vi "get all VIs in SciScan directory.vi"(7 "Path":path, 11 "keep GFG unlocked":bool) -> (3 "All Files in Dir":path[](array[path]))   [LabVIEW 2012]
doc: "SciScan 1.2 160622"
panel:
  out "size(s)":i32
  out "error out":errorcluster
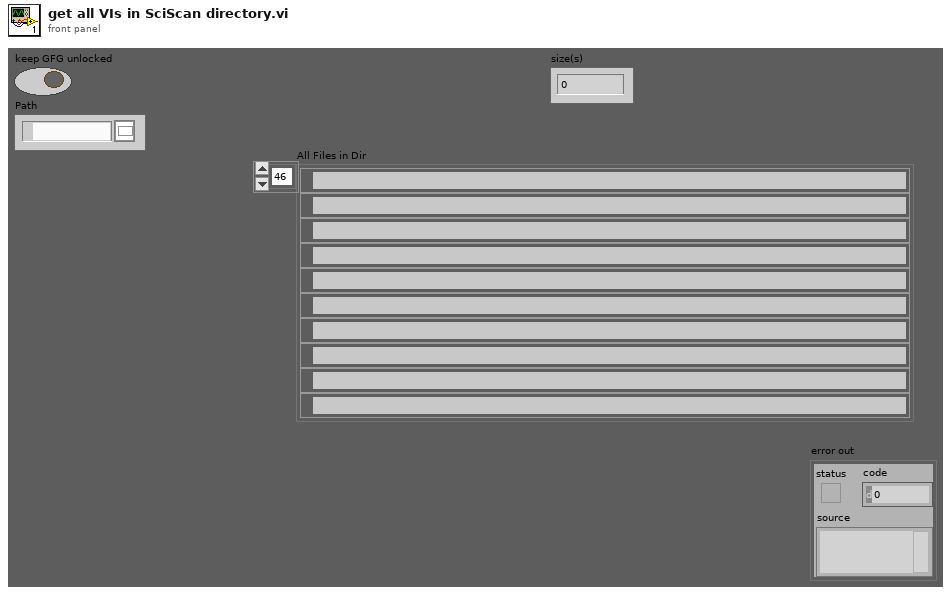
[diagram p1: front panel]
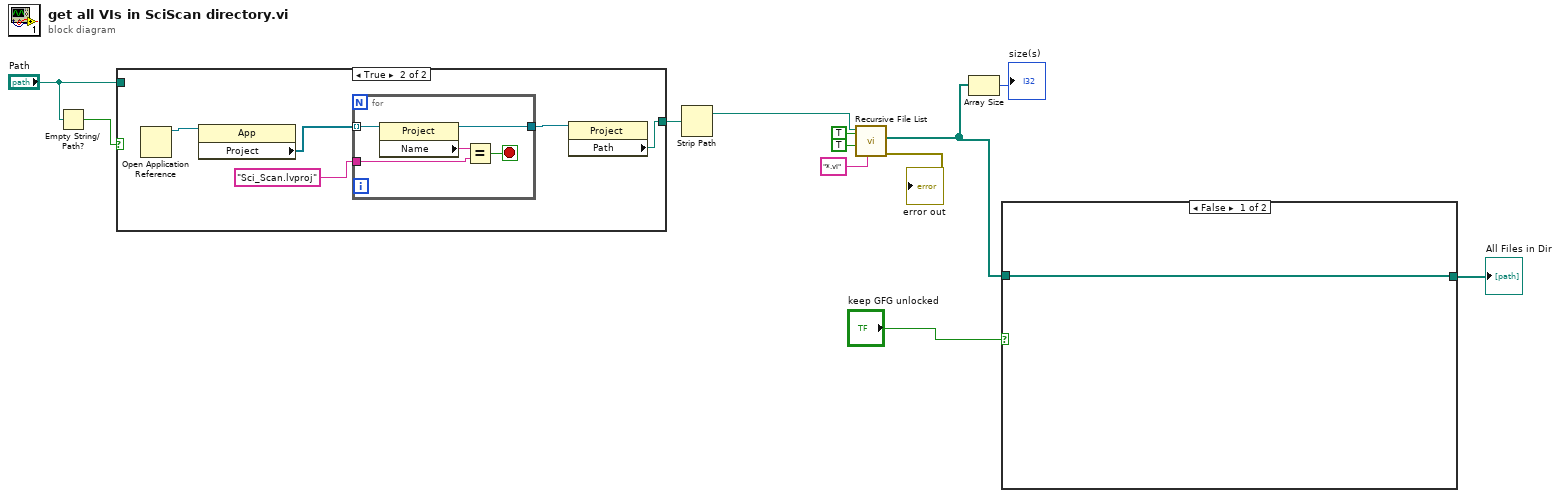
[diagram p0: block diagram]
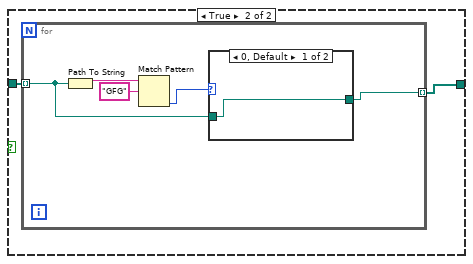
[diagram p3: hidden frame]
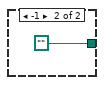
[diagram p4: hidden frame]
diagram:
  n1 = Empty String/Path?(string/path="Path") -> (empty?=w1:bool)
  n2 = case shown="True" w1 {
    tunnel: [w13 w14] -> w10
    tunnel: "Path" -> [w13 _]
    frame False {
    }
    frame True {
      n3 = Open Application Reference() -> (3:w18:refnum<vi>)  [unwired: 4 in, 1 out]
      n4 = property class="App"(reference=w18) -> ("Project"=w17:refnum<vi>[])  [unwired: 1 in, 2 out]
      n5 = for {
        tunnel: w17 -> [w23] mode=indexing
        tunnel: "Sci_Scan.lvproj" ("Name") -> [w21]
        tunnel: [w19] -> w15
        stop <- w20 stop-if-true
        n6 = property class="Project"(reference=w23) -> (reference out=w19:refnum<vi>, "Name"=w22:string)  [unwired: 1 in, 1 out]
        n7 = Equal?(x=w22, y=w21) -> (x = y?=w20:bool)
      }
      n8 = property class="Project"(reference=w15) -> ("Path"=w14:path)  [unwired: 1 in, 2 out]
    }
  }
  n9 = Strip Path(path=w10) -> (stripped path=w8:path)  [unwired: 1 out]
  n10 = call <vilib>:"Recursive File List.vi"("pattern"="*.vi", "Continue Recursing on Error? (F)"=TRUE, "Treat LLBs as Folders?"=TRUE, "Folder Path"=w8) -> ("error out"=→"error out":errorcluster, "All Files in Dir"=w5:path[])  [unwired: 3 in, 3 out]
  n11 = Array Size(array=w5) -> (size(s)=→"size(s)":i32)
  n12 = case shown="False" "keep GFG unlocked" {
    tunnel: w5 -> [w24 w26]
    tunnel: [w24 w25] -> w4
    frame False {
    }
    frame True {
      n13 = for {
        tunnel: w26 -> [w27] mode=indexing
        tunnel: [w28] -> w25 mode=indexing
        n14 = Path To String(path=w27) -> (string=w31:string)
        n15 = Match Pattern(string=w31, regular expression="GFG") -> (offset past match=w29:i32)  [unwired: 1 in, 3 out]
        n16 = case shown="0, Default" w29 {
          tunnel: [w32 path ""] -> w28
          tunnel: w27 -> [w32 _]
          frame 0, Default {
          }
          frame -1 {
          }
        }
      }
    }
  }
  "All Files in Dir" <- w4
